vi "Set Binning.vi"(8 "error in (no error)":errorcluster, 9 "dy":i32, 10 "dx":i32, 11 "Camera in":refnum<class "Camera.lvclass">) -> (0 "error out":errorcluster, 3 "Camera":refnum<class "Camera.lvclass">)   [LabVIEW 2020, in "Camera.lvclass"]
uses:
  Camera.lvclass
  Camera.lvclass/Camera.ctl
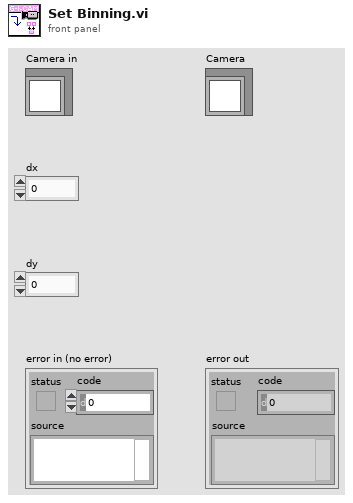
[diagram p1: front panel]
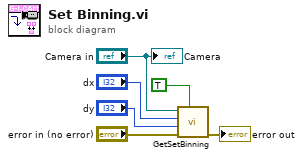
[diagram p0: block diagram]
diagram:
  n1 = call "GetSetBinning.vi"("Set?"=TRUE, "error in (no error)"="error in (no error)", "dy in"="dy", "dx in"="dx", "Camera in"="Camera in") -> ("error out"=→"error out":errorcluster)  [unwired: 4 in, 2 out]
  "Camera" <- "Camera in"
